vi "SUB-BLE Rx data (Mon)-Classify.vi"() -> (0 "data out":u8[](array[numeric]) format="%2x", 1 "Rx-set":bool, 2 "Rx-debug":bool, 3 "Rx-mon":bool, 4 "Packet No.":i32)   [LabVIEW 2015]
doc: "Use this template to create an application that executes repeatedly until you click the Stop button. This template polls the state of the Stop button and does not use events. Use the Top-Level Application template (not available in the Base package) to create a single-loop application with event handling."
uses:
  Global 1.vi
panel:
  out "BLE Packet (buf)":u8[](array[numeric])
  out "BLE Packet (data)":u8[](array[numeric])
  out "BLE Packet":bool=TRUE
  # "BLE 수신 데이터를 분류: Monitoring/Setting data"
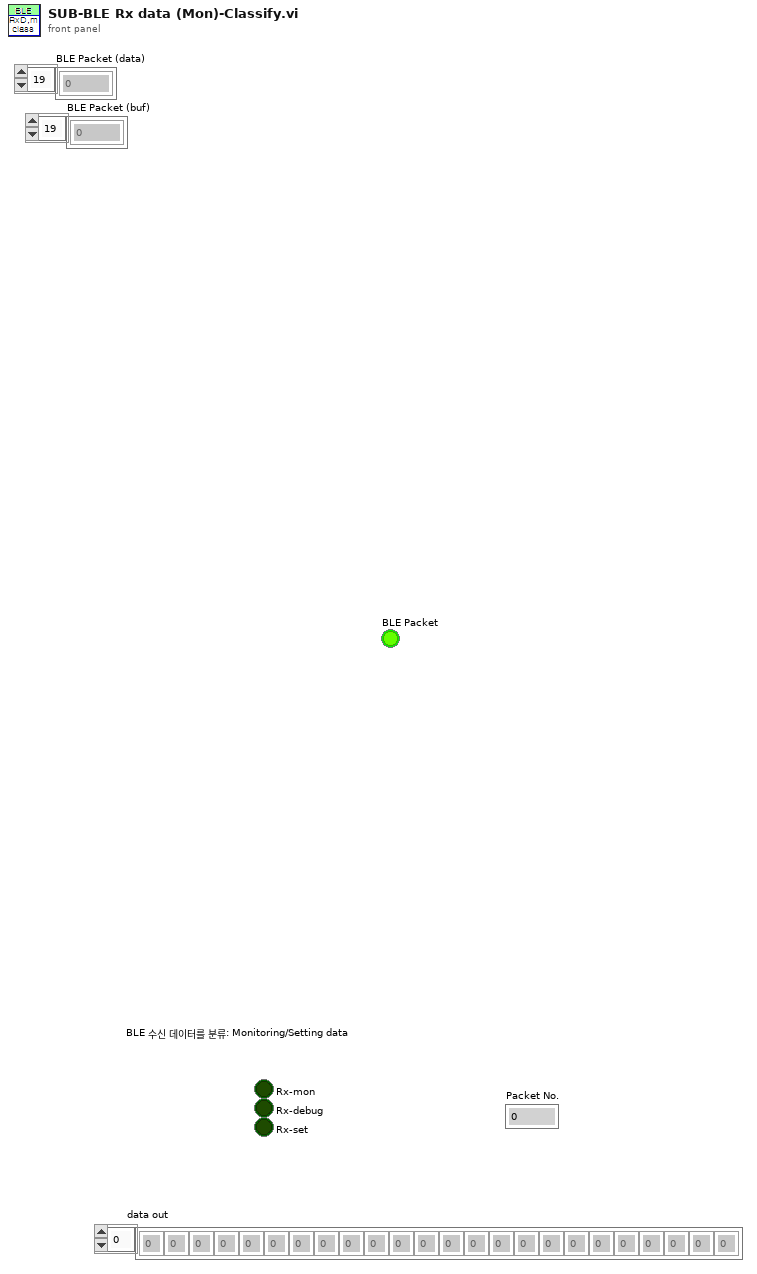
[diagram p1: front panel]
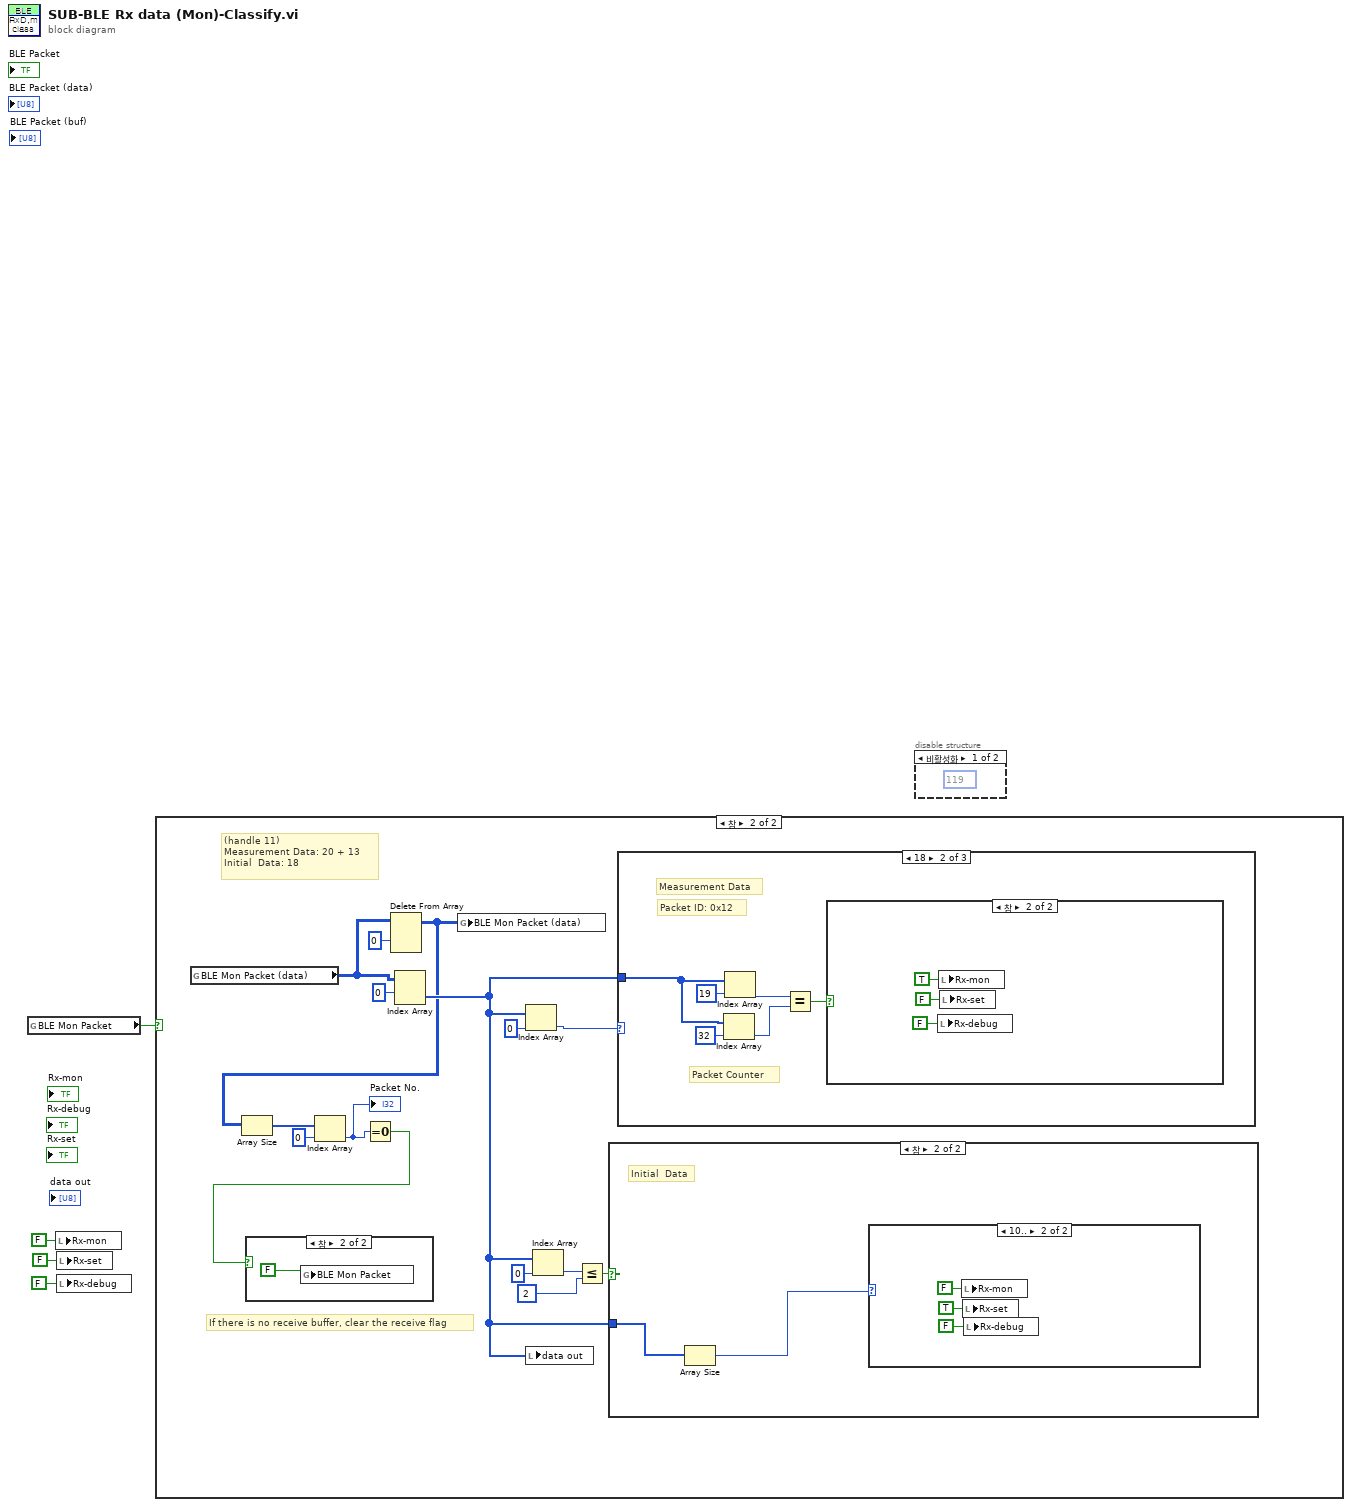
[diagram p0: block diagram]
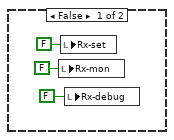
[diagram p3: hidden frame]
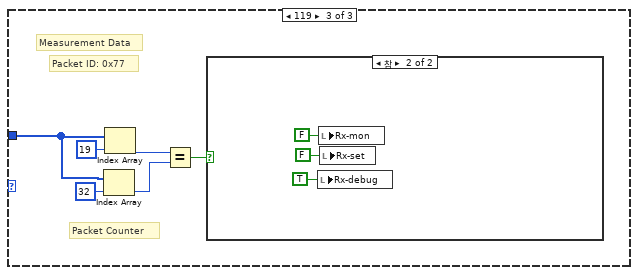
[diagram p9: hidden frame]
diagram:
  n1 = global read "Global 1.vi" "BLE Mon Packet"() -> (w4:bool)
  n2 = local write "Rx-mon"(FALSE ("Rx-mon")) -> ()
  n3 = local write "Rx-set"(FALSE ("Rx-set")) -> ()
  n4 = local write "Rx-debug"(FALSE ("Rx-set")) -> ()
  n5 = case shown="참" w4 {
    frame False {
      n6 = local write "Rx-mon"(FALSE ("Rx-mon")) -> ()
      n7 = local write "Rx-set"(FALSE ("Rx-set")) -> ()
      n8 = local write "Rx-debug"(FALSE ("Rx-set")) -> ()
    }
    frame True {
      # "(handle 11)\nMeasurement Data: 20 + 13\nInitial  Data: 18"
      # "If there is no receive buffer, clear the receive flag"
      n9 = global read "Global 1.vi" "BLE Mon Packet (data)"() -> (w15:u8[][])
      n10 = Delete From Array(array=w15, index (row)=0 ("인덱스 (행)")) -> (array with subset deleted=w13:u8[][])  [unwired: 2 in, 1 out]
      n11 = Array Size(array=w13) -> (size(s)=w12:i32[])
      n12 = Index Array(array=w12, index=0 ("인덱스")) -> (element=w10:i32)
      "Packet No." <- w10
      n13 = Equal To 0?(x=w10) -> (x = 0?=w9:bool)
      n14 = case shown="참" w9 {
        frame False {
        }
        frame True {
          n15 = global write "Global 1.vi" "BLE Mon Packet"(FALSE ("BLE Packet")) -> ()
        }
      }
      n16 = Index Array(array=w15, index (row)=0 ("인덱스 (행)")) -> (element=w16:u8[])  [unwired: 1 in]
      n17 = global write "Global 1.vi" "BLE Mon Packet (data)"(w13) -> ()
      n18 = Index Array(array=w16, index=0 ("인덱스")) -> (element=w8:u8)
      n19 = local write "data out"(w16) -> ()
      n20 = Index Array(array=w16, index=0 ("인덱스")) -> (element=w20:u8)
      n21 = Less Or Equal?(x=w20, y=2 ("인덱스")) -> (x <= y?=w18:bool)
      n22 = case shown="참" w18 {
        tunnel: w16 -> [_ w25]
        frame False {
        }
        frame True {
          # "Initial  Data"
          n23 = Array Size(array=w25) -> (size(s)=w24:i32)
          n24 = case shown="10.." w24 {
            frame 0, Default {
            }
            frame 10.. {
              n25 = local write "Rx-mon"(FALSE ("Rx-mon")) -> ()
              n26 = local write "Rx-set"(TRUE ("Rx-set")) -> ()
              n27 = local write "Rx-debug"(FALSE ("Rx-set")) -> ()
            }
          }
        }
      }
      n28 = case shown="18" w8 {
        tunnel: w16 -> [_ w30 w38]
        frame 0, Default {
        }
        frame 18 {
          # "Packet ID: 0x12"
          # "Measurement Data"
          # "Packet Counter"
          n29 = Index Array(array=w30, index=32 ("인덱스")) -> (element=w34:u8)
          n30 = Index Array(array=w30, index=19 ("인덱스")) -> (element=w33:u8)
          n31 = Equal?(x=w33, y=w34) -> (x = y?=w29:bool)
          n32 = case shown="참" w29 {
            frame False {
            }
            frame True {
              n33 = local write "Rx-debug"(FALSE ("Rx-set")) -> ()
              n34 = local write "Rx-mon"(TRUE ("Rx-mon")) -> ()
              n35 = local write "Rx-set"(FALSE ("Rx-set")) -> ()
            }
          }
        }
        frame 119 {
          # "Packet ID: 0x77"
          # "Measurement Data"
          # "Packet Counter"
          n36 = Index Array(array=w38, index=32 ("인덱스")) -> (element=w43:u8)
          n37 = Index Array(array=w38, index=19 ("인덱스")) -> (element=w42:u8)
          n38 = Equal?(x=w42, y=w43) -> (x = y?=w39:bool)
          n39 = case shown="참" w39 {
            frame False {
            }
            frame True {
              n40 = local write "Rx-debug"(TRUE ("Rx-set")) -> ()
              n41 = local write "Rx-mon"(FALSE ("Rx-mon")) -> ()
              n42 = local write "Rx-set"(FALSE ("Rx-set")) -> ()
            }
          }
        }
      }
    }
  }
  n43 = disable-structure shown="비활성화" {
    frame Disabled {
      (unwired) 119 ("인덱스")
    }
    frame Enabled {
    }
  }
